vi "Find optimal frequency.vi"(6 "Bottom end of range (GHz) (140.0)":dbl=140.0, 7 "Top end of range (GHz) (141.0)":dbl=141.0, 8 "Find optimal for negative polarization?":bool, 9 "C":dbl, 10 "Fit parameters":T2={"A"=0.572086, "S"=0.0835606, "M1"=140.286, "M2"=140.486}, 11 "Physical constants":T1={"T1e (s)"=0.03, "T1n (s)"=1500.0}) -> (3 "Optimal frequency (GHz)":dbl)   [LabVIEW 2015]
uses:
  Fit Parameters.ctl
  Physical Constants.ctl
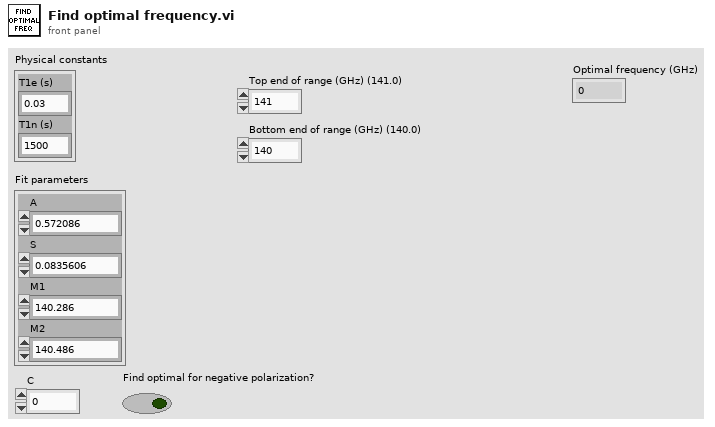
[diagram p1: front panel]
types:
  T1 = typedef "Physical Constants.ctl" = cluster{"T1e (s)":dbl, "T1n (s)":dbl}
  T2 = typedef "Fit Parameters.ctl" = cluster{"A":dbl, "S":dbl, "M1":dbl, "M2":dbl}
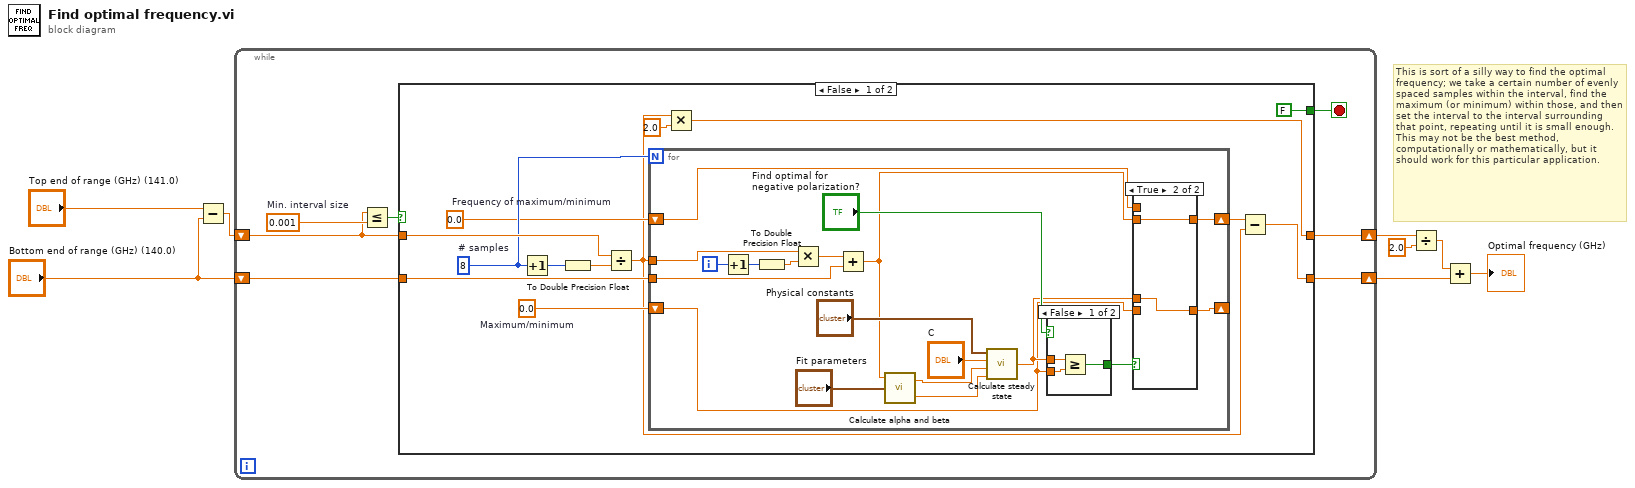
[diagram p0: block diagram]
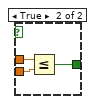
[diagram p3: hidden frame]
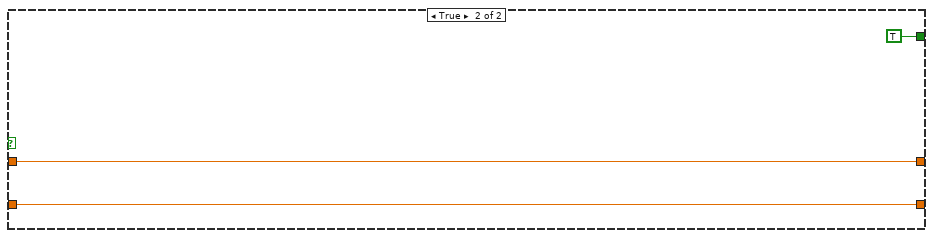
[diagram p4: hidden frame]
diagram:
  # "This is sort of a silly way to find the optimal frequency; we take a certain number of evenly spaced samples within the interval, find the maximum (or minimum) within those, and then set the interval to the interval surrounding that point, repeating until it is small enough.  This may not be the best method, computationally or mathematically, but it should work for this particular application."
  n1 = Subtract(x="Top end of range (GHz) (141.0)", y="Bottom end of range (GHz) (140.0)") -> (x-y=w6:dbl)
  n2 = while {
    shift-right: [w11] -> w5
    shift-left: w6 -> [w12]
    shift-right: [w9] -> w2
    shift-left: "Bottom end of range (GHz) (140.0)" -> [w10]
    stop <- w13 stop-if-true
    w15 = 0.001  # Min. interval size
    n3 = Less Or Equal?(x=w12, y=w15) -> (x <= y?=w14:bool)
    n4 = case shown="False" w14 {
      tunnel: [FALSE TRUE] -> w13
      tunnel: w12 -> [w27 w58]
      tunnel: [w22 w58] -> w11
      tunnel: w10 -> [w19 w59]
      tunnel: [w16 w59] -> w9
      frame False {
        w20 = 0.0  # Maximum/minimum
        w21 = 0.0  # Frequency of maximum/minimum
        w24 = 8  # # samples
        n5 = Increment(x=w24) -> (x+1=w25:i32)
        n6 = To Double Precision Float(number=w25) -> (double precision float=w26:dbl)
        n7 = Divide(x=w27, y=w26) -> (x/y=w17:dbl)
        n8 = for {
          N: w24 -> [_]
          tunnel: w17 -> [w46]
          shift-right: [w32] -> w18
          shift-left: w21 -> [w30]
          shift-right: [w31] -> _
          shift-left: w20 -> [w29]
          tunnel: w19 -> [w34]
          i -> [w44]
          n9 = Increment(x=w44) -> (x+1=w45:i32)
          n10 = To Double Precision Float(number=w45) -> (double precision float=w47:dbl)
          n11 = Multiply(x=w46, y=w47) -> (x*y=w35:dbl)
          n12 = Add(x=w35, y=w34) -> (x+y=w33:dbl)
          n13 = call "Calculate alpha and beta.vi"("Fit parameters"="Fit parameters", "Frequency (GHz)"=w33) -> ("Beta"=w40:dbl, "Alpha"=w41:dbl)  [unwired: 1 in]
          n14 = call "Calculate steady state.vi"("Beta"=w40, "Alpha"=w41, "C"="C", "Physical constants"="Physical constants") -> ("Steady state"=w36:dbl)
          n15 = case shown="False" "Find optimal for negative polarization?" {
            tunnel: w36 -> [w54 w57]
            tunnel: w29 -> [w53 w56]
            tunnel: [w52 w55] -> w37
            frame False {
              n16 = Greater Or Equal?(x=w54, y=w53) -> (x >= y?=w52:bool)
            }
            frame True {
              n17 = Less Or Equal?(x=w57, y=w56) -> (x <= y?=w55:bool)
            }
          }
          n18 = case shown="True" w37 {
            tunnel: w36 -> [_ w50]
            tunnel: w33 -> [_ w51]
            tunnel: [w49 w51] -> w32
            tunnel: [w48 w50] -> w31
            tunnel: w30 -> [w49 _]
            tunnel: w29 -> [w48 _]
            frame False {
            }
            frame True {
            }
          }
        }
        n19 = Multiply(x=w17, y=2.0) -> (x*y=w22:dbl)
        n20 = Subtract(x=w18, y=w17) -> (x-y=w16:dbl)
      }
      frame True {
      }
    }
  }
  n21 = Divide(x=w5, y=2.0) -> (x/y=w3:dbl)
  n22 = Add(x=w3, y=w2) -> (x+y=→"Optimal frequency (GHz)":dbl)
